vi "Get Group Metadata.vi"(0 "reference in":refnum<class "TDMS_DataHandler.lvclass">, 5 "error in (no error)":errorcluster) -> (14 "reference out":refnum<class "TDMS_DataHandler.lvclass">, 16 "Tdms metadata out":T1, 19 "error out":errorcluster)   [LabVIEW 2019, in "TDMS_DataHandler.lvclass"]
uses:
  TDMS_DataHandler.lvclass
  Fcurve Meta data.ctl
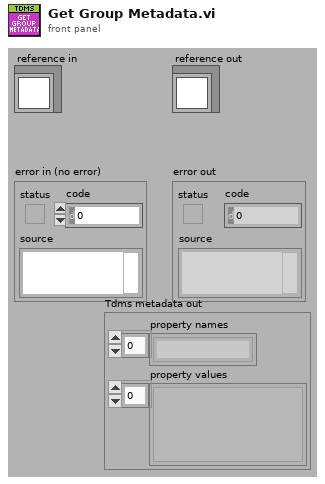
[diagram p1: front panel]
types:
  T1 = cluster{"property names":string[], "property values":variant[]}
  T2 = typedef "TDMS_DataHandler.lvclass/Fcurve Meta data.ctl" = cluster{"property names":string[], "property values":variant[]}
  T3 = typedef "TDMS_DataHandler.lvclass/ObjectAttributesRef.ctl" = refnum<data-value>
  T4 = typedef "TDMS_DataHandler.lvclass/ObjectAttributes.ctl" = cluster{"Directory":path, "FilePath":path, "FileRef":refnum<k34>, "ExperimentName":string, "GroupName":string, "ChannelNames":string[], "Datum":waveform(dbl)[], "Group_Metadata":cluster{"property names":string[], "property values":variant[]}, "Channel_Metadata":cluster{"property names":string[], "property values":variant[]}}
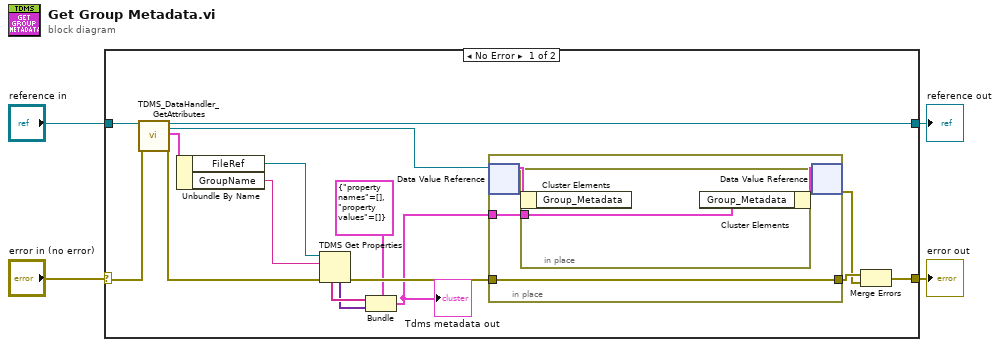
[diagram p0: block diagram]
diagram:
  n1 = case shown="No Error" "error in (no error)" {
    selector: "error in (no error)" -> [w17 w27]
    tunnel: [w20 w27] -> w3
    tunnel: [w18 w26] -> w1
    tunnel: "reference in" -> [w19 w26]
    frame No Error {
      n2 = call "TDMS_DataHandler_GetAttributes.vi"("reference in"=w19, "error in (no error)"=w17) -> ("reference out"=w18:refnum<class "TDMS_DataHandler.lvclass">, "attributes ref"=w13:T3, "attributes"=w16:T4, "error out"=w11:errorcluster)  [unwired: 14 in]
      n3 = Unbundle By Name(w16) -> ("FileRef"=w12:refnum<k34>, "GroupName"=w5:string)
      n4 = TDMS Get Properties(8:w11, 10:w5, 11:w12) -> (0:w10:errorcluster, 4:w8:variant[], 6:w9:string[])  [unwired: 3 in, 3 out]
      n5 = Bundle(cluster=T2 {"property names"=[], "property values"=[]} ("Fcurve Metadata"), "property names"=w9, "property values"=w8) -> (w6:T2)
      "Tdms metadata out" <- w6
      n6 = in-place {
        in-place-border: w10 -> [w22]
        in-place-border: [w22] -> w15
        in-place-border: w6 -> [w21]
        n7 = in-place-dvr #1(w13) -> (w23:T4)  [unwired: 1 out]
        n8 = in-place {
          in-place-border: w21 -> [w25]
          n9 = in-place-cluster #2(w23) -> ()  [unwired: 1 out]
          n10 = in-place-cluster #2("Group_Metadata"=w25) -> (w24:T4)
        }
        n11 = in-place-dvr #1(w24) -> (w14:errorcluster)  [unwired: 1 out]
      }
      n12 = Merge Errors(w15, w14) -> (w20:errorcluster)
    }
    frame Error {
    }
  }
  "error out" <- w3
  "reference out" <- w1
